vi "CohortDisplay.vi"(8 "error in (no error)":errorcluster, 10 "Cohort Ref":refnum<vi>, 11 "Cohort in":refnum<class "Cohort.lvclass">) -> (0 "error out":errorcluster, 3 "Cohort out":refnum<class "Cohort.lvclass">)   [LabVIEW 2012, in "Cohort.lvclass"]
uses:
  Cohort.lvclass
  CohortConfig.ctl
  UserControl/LeftPanel.ctl
  UserControl/ElectdPanel.ctl
  UserControl/ElectdTerminal.ctl
  Cohort.lvclass/Cohort.ctl
  StimulCtrls.lvlib
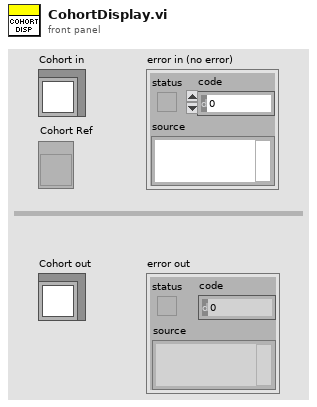
[diagram p1: front panel]
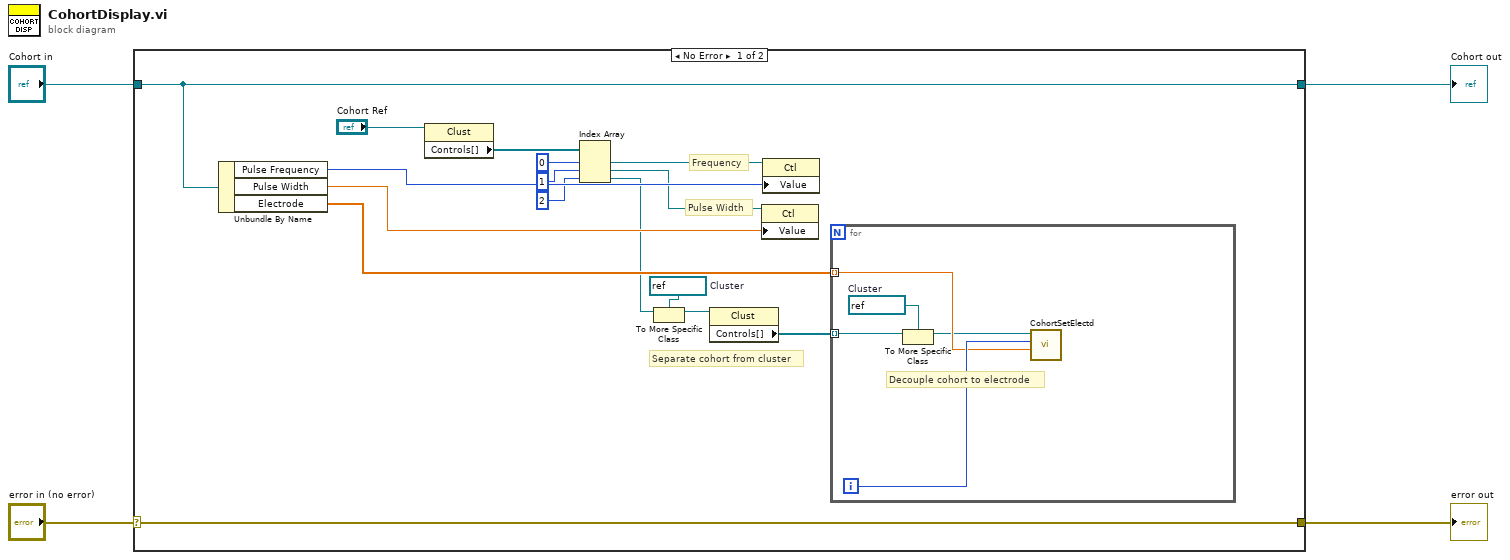
[diagram p0: block diagram]
diagram:
  n1 = case shown="No Error" "error in (no error)" {
    selector: "error in (no error)" -> [w20 w26]
    tunnel: [w20 w26] -> w3
    tunnel: [w19 w27] -> w1
    tunnel: "Cohort in" -> [w19 w27]
    frame No Error {
      w7 = refnum<vi> refnum  # Cluster
      # "Separate cohort from cluster"
      # "Pulse Width"
      # "Frequency"
      n2 = Unbundle By Name(w19) -> ("Pulse Frequency"=w12:u8, "Pulse Width"=w8:sgl, "Electrode"=w18:sgl[])
      n3 = property class="Clust"(reference="Cohort Ref") -> ("Controls[]"=w15:refnum<vi>[])  [unwired: 1 in, 2 out]
      n4 = Index Array(array=w15, index #1=0 ("index"), index #2=1 ("index"), index #3=2 ("index")) -> (element #1=w13:refnum<vi>, element #2=w9:refnum<vi>, element #3=w5:refnum<vi>)
      n5 = To More Specific Class(target class=w7, reference=w5) -> (specific class reference=w6:refnum<vi>)  [unwired: 1 in, 1 out]
      n6 = property class="Clust"(reference=w6) -> ("Controls[]"=w17:refnum<vi>[])  [unwired: 1 in, 2 out]
      n7 = property class="Ctl"(reference=w9, "Value"=w8) -> ()  [unwired: 1 in, 2 out]
      n8 = property class="Ctl"(reference=w13, "Value"=w12) -> ()  [unwired: 1 in, 2 out]
      n9 = for {
        tunnel: w18 -> [w24] mode=indexing
        tunnel: w17 -> [w23] mode=indexing
        i -> [w25]
        w21 = refnum<vi> refnum  # Cluster
        # "Decouple cohort to electrode"
        n10 = To More Specific Class(target class=w21, reference=w23) -> (specific class reference=w22:refnum<vi>)  [unwired: 1 in, 1 out]
        n11 = call "CohortSetElectd.vi"("Electd Ref"=w22, "Index"=w25, "Amplitude"=w24) -> ()  [unwired: 8 in]
      }
    }
    frame Error {
    }
  }
  "error out" <- w3
  "Cohort out" <- w1
